vi "Registrar-Usuarios-V3.vi"() -> ()   [LabVIEW 2024]
uses:
  <vilib>/Utility/file.llb/Read Delimited Spreadsheet (string).vi
  <vilib>/Utility/file.llb/Write Delimited Spreadsheet (string).vi
panel:
  out "Path":path=path "C:/Users/willi/GITHUB/TG/OBJ 2 - RECOLECCION DE DATOS/registro-usuarios.csv"
  out "ActualUser":i32
  out "Array 2":i32[](array[numeric])
  out "Array":T1(array[cluster])
  in  "Tab Control":enum32{"Seleccionar ", "Registrar"}(tab)
  in  "Registrar Usuario":T2 {"Edad" format="%#_13g"}
  in  "registrButt":bool
  in  "stop":bool
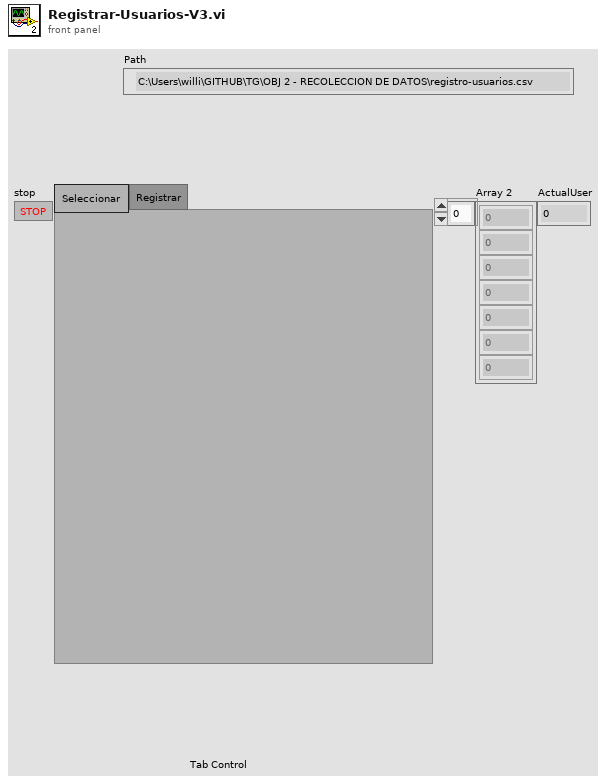
[diagram p1: front panel]
types:
  T1 = cluster{"Número Usuario":string, "Edad":string, "Genero":enum16{"Male", "Female"}, "Hipermetropia":enum16{"No", "Si"}, "Miopia":enum16{"No", "Si"}}[]
  T2 = cluster{"Genero":enum16{"Male", "Female"}, "Edad":dbl, "Hipermetropia":enum16{"No", "Si"}, "Miopia":enum16{"No", "Si"}}
  T3 = cluster{"Número Usuario":string, "Edad":string, "Genero":enum16{"Male", "Female"}, "Hipermetropia":enum16{"No", "Si"}, "Miopia":enum16{"No", "Si"}}
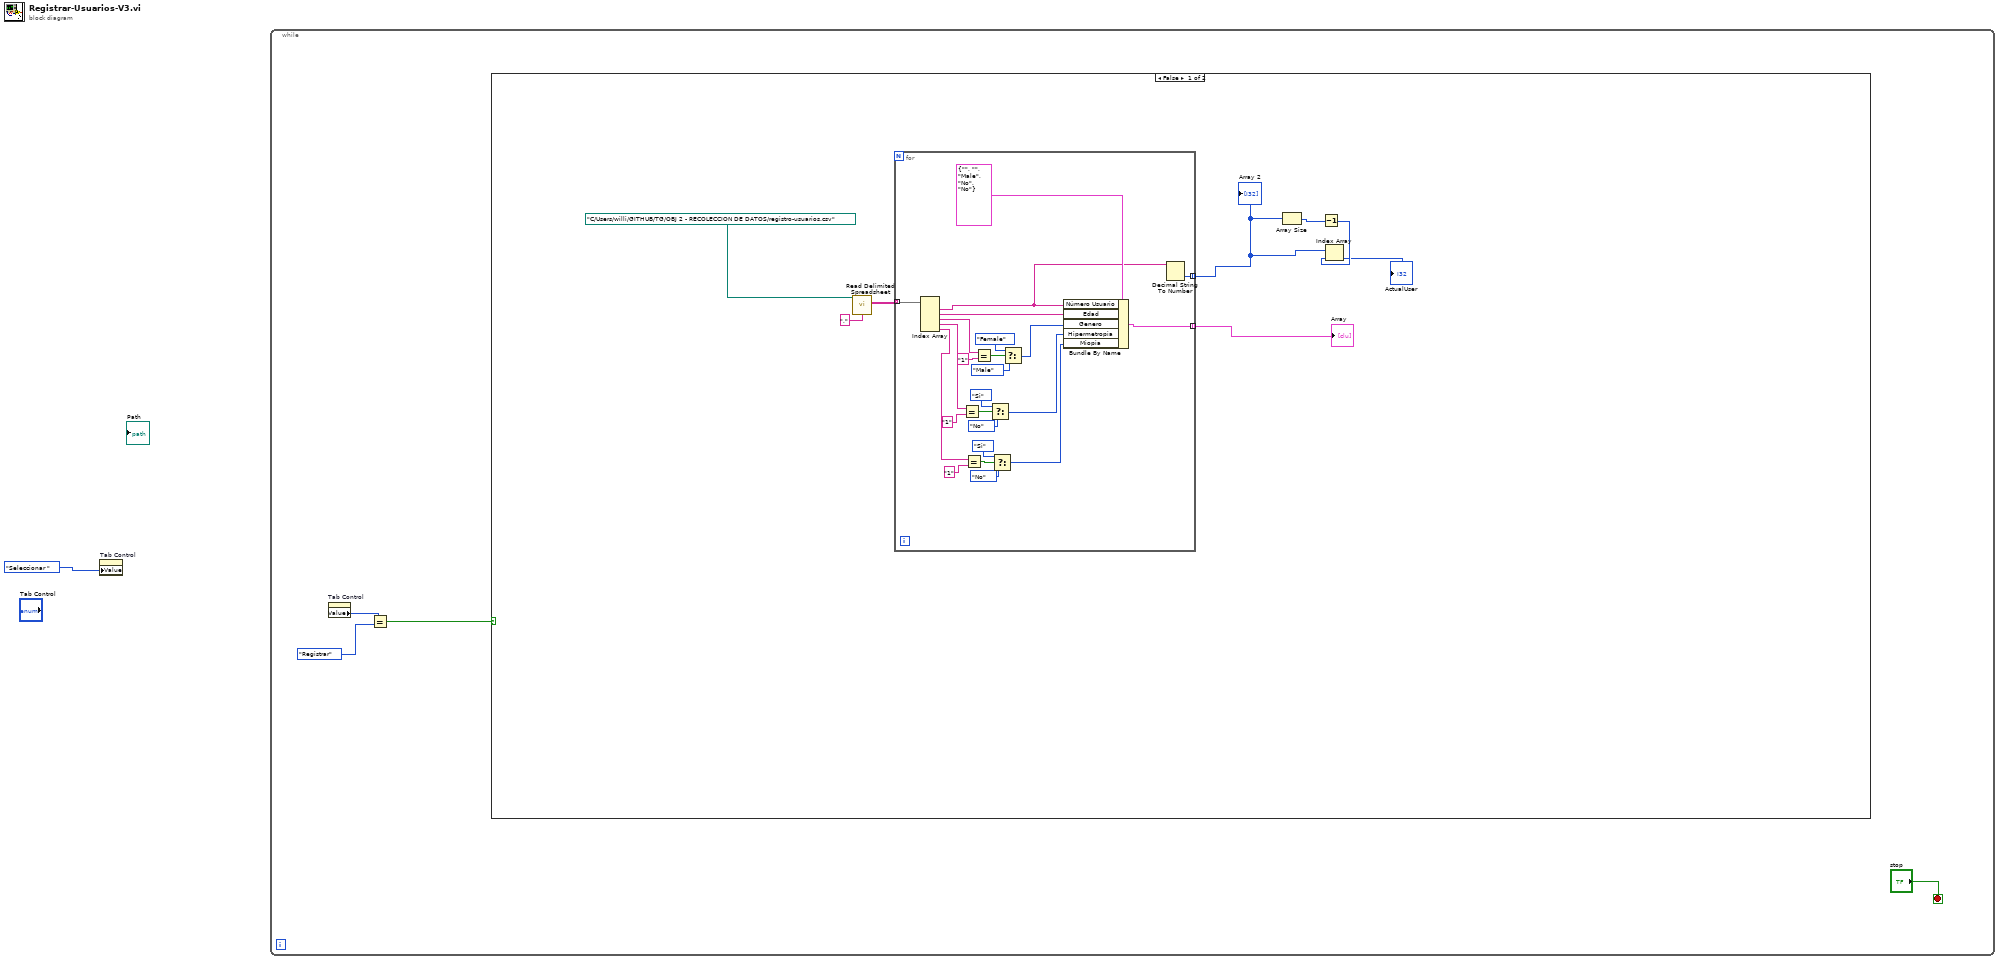
[diagram p0: block diagram]
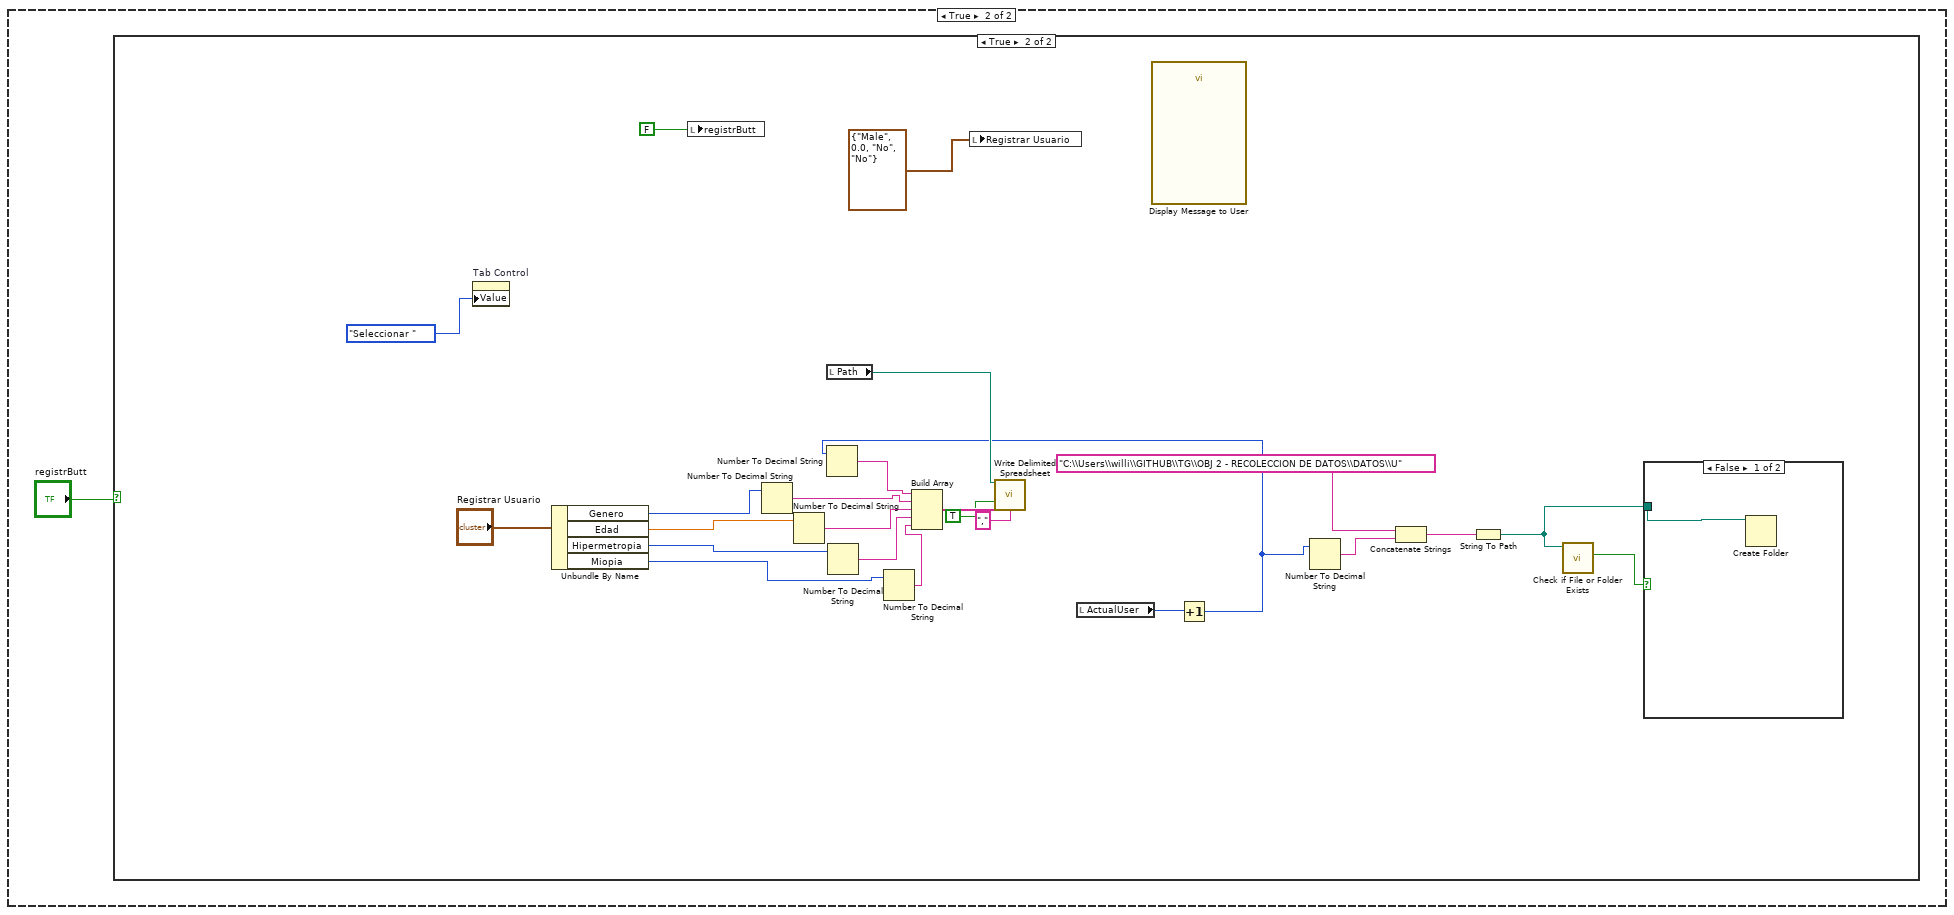
[diagram p2: hidden frame]
diagram:
  n1 = property on="Tab Control" class="TabCtl (strict)"("Value"=enum32{"Seleccionar ", "Registrar"}."Seleccionar " ("Tab Control")) -> ()  [unwired: 2 in, 2 out]
  n2 = while {
    stop <- "stop" stop-if-true
    n3 = property on="Tab Control" class="TabCtl (strict)"() -> ("Value"=w4:enum32{"Seleccionar ", "Registrar"})  [unwired: 2 in, 2 out]
    n4 = Equal?(x=w4, y=enum32{"Seleccionar ", "Registrar"}."Registrar" ("Tab Control")) -> (x = y?=w2:bool)
    n5 = case shown="False" w2 {
      frame False {
        n6 = call-poly <vilib>:"Read Delimited Spreadsheet.vi"("file path (dialog if empty)"=path "C:/Users/willi/GITHUB/TG/OBJ 2 - RECOLECCION DE DATOS/registro-usuarios.csv", "delimiter (\\t)"="," ("delimiter (\\t)")) -> ("all rows"=w12:string[][])  [unwired: 8 in, 5 out]
        n7 = for {
          tunnel: w12 -> [w37] mode=indexing
          tunnel: [w16] -> w11 mode=indexing
          tunnel: [w14] -> w9 mode=indexing
          n8 = Index Array(array=w37) -> (element #1=w15:string, element #2=w35:string, element #3=w33:string, element #4=w24:string, element #5=w18:string)  [unwired: 5 in]
          n9 = Equal?(x=w24, y="1") -> (x = y?=w27:bool)
          n10 = Equal?(x=w18, y="1") -> (x = y?=w21:bool)
          n11 = Equal?(x=w33, y="1") -> (x = y?=w32:bool)
          n12 = Select(t=enum16{"No", "Si"}."Si" ("Hipermetropia"), s=w27, f=enum16{"No", "Si"}."No" ("Hipermetropia")) -> (s? t:f=w23:enum16{"No", "Si"})
          n13 = Select(t=enum16{"No", "Si"}."Si" ("Hipermetropia"), s=w21, f=enum16{"No", "Si"}."No" ("Hipermetropia")) -> (s? t:f=w17:enum16{"No", "Si"})
          n14 = Select(t=enum16{"Male", "Female"}."Female" ("Genero"), s=w32, f=enum16{"Male", "Female"}."Male" ("Genero")) -> (s? t:f=w29:enum16{"Male", "Female"})
          n15 = Bundle By Name(cluster=T3 {"Número Usuario"="", "Edad"="", "Genero"=enum."Male", "Hipermetropia"=enum."No", "Miopia"=enum."No"} ("Registrar Usuario"), "Número Usuario"=w15, "Edad"=w35, "Genero"=w29, "Hipermetropia"=w23, "Miopia"=w17) -> (w16:T3)
          n16 = Decimal String To Number(string=w15) -> (number=w14:i32)  [unwired: 2 in, 1 out]
        }
        "Array" <- w11
        "Array 2" <- w9
        n17 = Array Size(array=w9) -> (size(s)=w8:i32)
        n18 = Decrement(x=w8) -> (x-1=w7:i32)
        n19 = Index Array(array=w9, index=w7) -> (element=→"ActualUser":i32)
      }
      frame True {
        n20 = case shown="True" "registrButt" {
          frame False {
          }
          frame True {
            n21 = property on="Tab Control" class="TabCtl (strict)"("Value"=enum32{"Seleccionar ", "Registrar"}."Seleccionar " ("Tab Control")) -> ()  [unwired: 2 in, 2 out]
            n22 = Unbundle By Name("Registrar Usuario") -> ("Genero"=w52:enum16{"Male", "Female"}, "Edad"=w51:dbl, "Hipermetropia"=w50:enum16{"No", "Si"}, "Miopia"=w49:enum16{"No", "Si"})
            n23 = local write "registrButt"(FALSE) -> ()
            n24 = Number To Decimal String(number=w52) -> (decimal integer string=w53:string)  [unwired: 1 in]
            n25 = Number To Decimal String(number=w51) -> (decimal integer string=w56:string)  [unwired: 1 in]
            n26 = local read "Path"() -> (w45:path)
            n27 = Number To Decimal String(number=w50) -> (decimal integer string=w57:string)  [unwired: 1 in]
            n28 = Number To Decimal String(number=w49) -> (decimal integer string=w58:string)  [unwired: 1 in]
            n29 = local write "Registrar Usuario"(T2 {"Genero"=enum."Male", "Edad"=0.0, "Hipermetropia"=enum."No", "Miopia"=enum."No"} ("Registrar Usuario")) -> ()
            n30 = local read "ActualUser"() -> (w40:i32)
            n31 = call "Display Message to User"() -> ()  [unwired: 10 in, 2 out]
            n32 = Increment(x=w40) -> (x+1=w39:i32)
            n33 = Number To Decimal String(number=w39) -> (decimal integer string=w48:string)  [unwired: 1 in]
            n34 = Build Array(w48, w53, w56, w57, w58) -> (w61:string[])
            n35 = call-poly <vilib>:"Write Delimited Spreadsheet.vi"("file path (dialog if empty)"=w45, "1D data"=w61, "append to file? (new file:F)"=TRUE, "delimiter (\\t)"="," ("delimiter (\\t)")) -> ()  [unwired: 10 in, 2 out]
            n36 = Number To Decimal String(number=w39) -> (decimal integer string=w47:string)  [unwired: 1 in]
            n37 = Concatenate Strings("C:\\Users\\willi\\GITHUB\\TG\\OBJ 2 - RECOLECCION DE DATOS\\DATOS\\U" ("string"), w47) -> (w44:string)
            n38 = String To Path(string=w44) -> (path=w42:path)
            n39 = call <vilib>:"Check if File or Folder Exists.vi"("path"=w42) -> ("file or folder exists?"=w43:bool)  [unwired: 8 in, 2 out]
            n40 = case shown="False" w43 {
              tunnel: w42 -> [w63 _]
              frame False {
                n41 = Create Folder(path (use dialog)=w63) -> ()  [unwired: 2 in, 3 out]
              }
              frame True {
              }
            }
          }
        }
      }
    }
  }
